vi "ZAlign_Error_Clusters.vi"(7 "FilterCtrls[]":refnum<vi>[](array[refnum]), 8 "Error in":errorcluster, 10 "ConPane":refnum<vi>, 11 "Panel":refnum<vi>) -> (0 "Error out":errorcluster, 2 "Width":u32, 3 "Height":u32)   [LabVIEW 2014, in "ZAlign.lvlib"]
doc: "ZAlign.lvlib:ZAlign_Error_Clusters.vi\n----------------------------------------------\nBottom align Error Clusters \n\nInputs:\n---------------------\n- Error in : Cluster; \n- ConPane : Refnum; \n- Panel : Refnum; \n\nOutputs:\n---------------------\n- Error out : Cluster; \n- Width : U32; \n- Height : U32; \n\n----------------------------------------------\n16/03/2015\nZühlke Engineering AG\nCH-8952 Schlieren\nwww.zuehlke.com"
uses:
  ZAlign.lvlib
panel:
  # "Connector Pane"
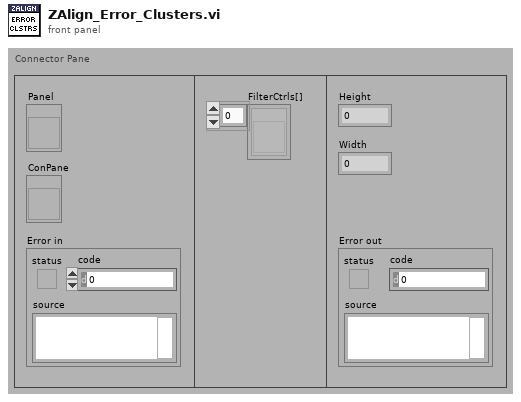
[diagram p1: front panel]
types:
  T1 = typedef "LVRectTypeDef.ctl" = cluster{"Left":i16, "Top":i16, "Right":i16, "Bottom":i16}
  T2 = enum32{"Top Edges", "Vertical Centers", "Bottom Edges", "Left Edges", "Horizontal Centers", "Right Edges"}
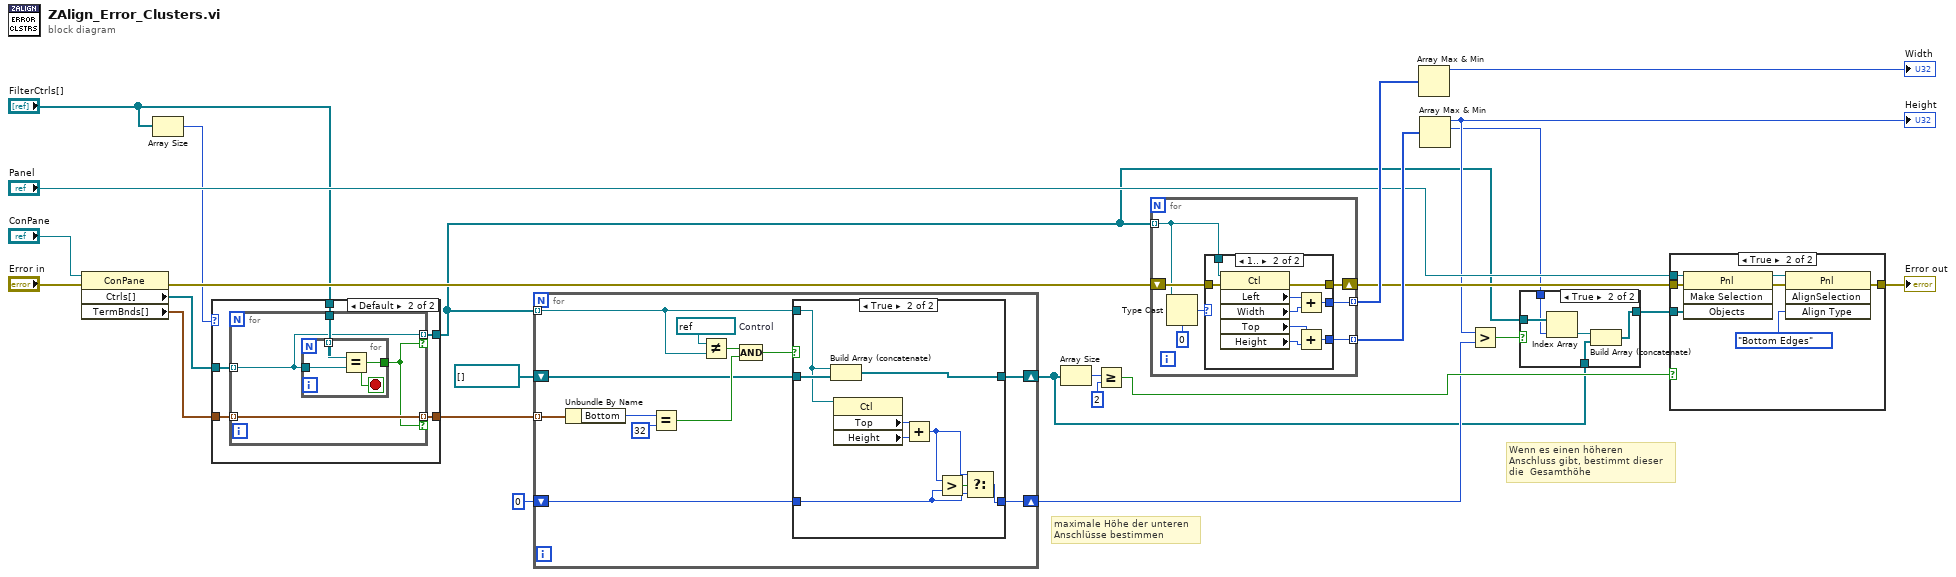
[diagram p0: block diagram]
diagram:
  # "Wenn es einen höheren\nAnschluss gibt, bestimmt dieser \ndie  Gesamthöhe"
  # "maximale Höhe der unteren \nAnschlüsse bestimmen"
  n1 = property class="ConPane"(reference="ConPane", error in="Error in") -> (error out=w17:errorcluster, "Ctrls[]"=w2:refnum<vi>[], "TermBnds[]"=w6:T1[])  [unwired: 1 out]
  n2 = Array Size(array="FilterCtrls[]") -> (size(s)=w4:i32)
  n3 = case shown="Default" w4 {
    tunnel: w2 -> [w28 w33]
    tunnel: [w28 w32] -> w1
    tunnel: "FilterCtrls[]" -> [_ w31]
    tunnel: w6 -> [w27 w30]
    tunnel: [w27 w29] -> w5
    frame 0 {
    }
    frame Default {
      n4 = for {
        tunnel: w33 -> [w36] mode=indexing
        tunnel: w31 -> [w37]
        tunnel: [w36] -> w32 mode=indexing if=w34
        tunnel: w30 -> [w35] mode=indexing
        tunnel: [w35] -> w29 mode=indexing if=w34
        n5 = for {
          tunnel: w36 -> [w40]
          tunnel: w37 -> [w39] mode=indexing
          tunnel: [w38] -> w34
          stop <- w38 stop-if-true
          n6 = Equal?(x=w39, y=w40) -> (x = y?=w38:bool)
        }
      }
    }
  }
  n7 = for {
    tunnel: w1 -> [w41] mode=indexing
    tunnel: w5 -> [w44] mode=indexing
    shift-right: [w49] -> w8
    shift-left: refnum<vi>[] [] -> [w45]
    shift-right: [w42] -> w11
    shift-left: u32 0 -> [w43]
    w47 = refnum<vi> refnum  # Control
    n8 = Unbundle By Name(w44) -> ("Bottom"=w52:i16)
    n9 = Equal?(x=w52, y=i16 32) -> (x = y?=w50:bool)
    n10 = Not Equal?(x=w47, y=w41) -> (x != y?=w48:bool)
    n11 = Compound Arithmetic op=AND(w48, w50) -> (w46:bool)
    n12 = case shown="True" w46 {
      tunnel: w41 -> [_ w59]
      tunnel: [w54 w63] -> w49
      tunnel: w45 -> [w54 w62]
      tunnel: w43 -> [w53 w55]
      tunnel: [w53 w56] -> w42
      frame False {
      }
      frame True {
        n13 = Build Array (concatenate)(w59, w62) -> (w63:refnum<vi>[])
        n14 = property class="Ctl"(reference=w59) -> ("Top"=w61:i32, "Height"=w60:u32)  [unwired: 1 in, 2 out]
        n15 = Add(x=w61, y=w60) -> (x+y=w57:u32)
        n16 = Greater?(x=w57, y=w55) -> (0:w58:bool)
        n17 = Select(t=w57, s=w58, f=w55) -> (s? t:f=w56:u32)
      }
    }
  }
  n18 = Array Size(array=w8) -> (size(s)=w20:i32)
  n19 = Greater Or Equal?(x=w20, y=2) -> (x >= y?=w14:bool)
  n20 = for {
    tunnel: w1 -> [w65] mode=indexing
    tunnel: [w68] -> w23 mode=indexing
    tunnel: [w67] -> w21 mode=indexing
    shift-right: [w69] -> w16
    shift-left: w17 -> [w70]
    n21 = Type Cast(type=u64 0, x=w65) -> (*(type *) &x=w66:u64)
    n22 = case shown="1.." w66 {
      tunnel: w70 -> [w71 w80]
      tunnel: [w71 w79] -> w69
      tunnel: [_ w74] -> w68
      tunnel: [_ w73] -> w67
      tunnel: w65 -> [_ w72]
      frame 0, Default {
      }
      frame 1.. {
        n23 = property class="Ctl"(reference=w72, error in=w80) -> (error out=w79:errorcluster, "Left"=w78:i32, "Width"=w77:u32, "Top"=w76:i32, "Height"=w75:u32)  [unwired: 1 out]
        n24 = Add(x=w78, y=w77) -> (x+y=w74:u32)
        n25 = Add(x=w76, y=w75) -> (x+y=w73:u32)
      }
    }
  }
  n26 = Array Max & Min(array=w23) -> (max value=→"Width":u32)  [unwired: 3 out]
  n27 = Array Max & Min(array=w21) -> (max value=w12:u32, max index (indices)=w9:i32)  [unwired: 2 out]
  "Height" <- w12
  n28 = Greater?(x=w12, y=w11) -> (0:w10:bool)
  n29 = case shown="True" w10 {
    tunnel: w1 -> [_ w86]
    tunnel: w9 -> [_ w85]
    tunnel: w8 -> [w81 w83]
    tunnel: [w81 w82] -> w7
    frame False {
    }
    frame True {
      n30 = Index Array(array=w86, index=w85) -> (element=w84:refnum<vi>)
      n31 = Build Array (concatenate)(w84, w83) -> (w82:refnum<vi>[])
    }
  }
  n32 = case shown="True" w14 {
    tunnel: "Panel" -> [_ w94]
    tunnel: w16 -> [w87 w93]
    tunnel: w7 -> [_ w92]
    tunnel: [w87 w91] -> w15
    frame False {
    }
    frame True {
      n33 = invoke class="Pnl" method="Make Selection"(reference=w94, error in=w93, "Objects"=w92) -> (reference out=w88:refnum<vi>, error out=w90:errorcluster)  [unwired: 1 in, 2 out]
      n34 = invoke class="Pnl" method="AlignSelection"(reference=w88, error in=w90, "Align Type"=T2."Bottom Edges") -> (error out=w91:errorcluster)  [unwired: 1 in, 3 out]
    }
  }
  "Error out" <- w15
